vi "Debug Settings FG.vi"(8 "error in (no error)":errorcluster, 10 "Debug Settings In":T2, 11 "Operation":T1) -> (0 "error out":errorcluster, 2 "Debug Settings Out":T2)   [LabVIEW 2013]
uses:
  Debug Settings Cluster.ctl
  Debug Settings FG Enum.ctl
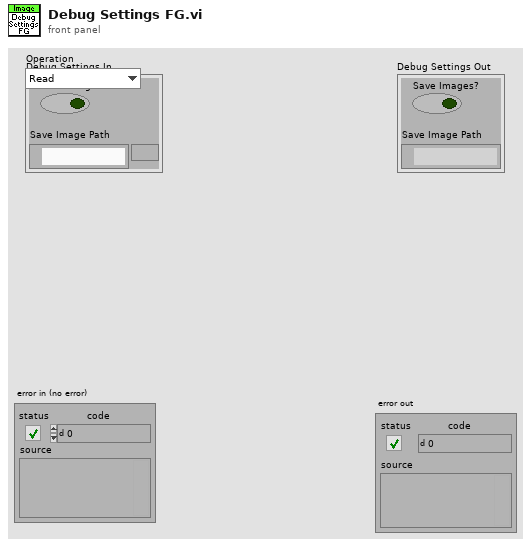
[diagram p1: front panel]
types:
  T1 = typedef "Debug Settings FG Enum.ctl" = enum16{"Read", "Write"}
  T2 = typedef "Debug Settings Cluster.ctl" = cluster{"Save Images?":bool, "Save Image Path":path}
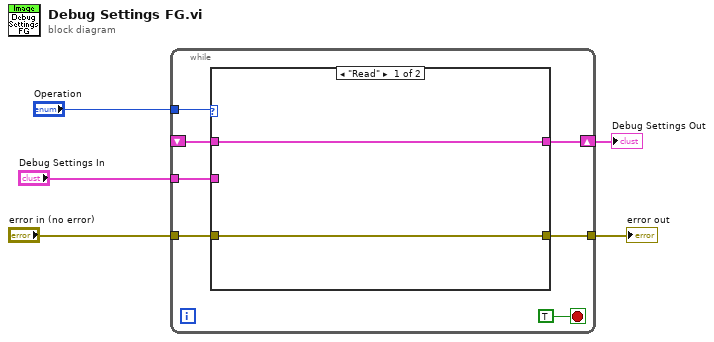
[diagram p0: block diagram]
diagram:
  n1 = while {
    tunnel: "Operation" -> [w11]
    tunnel: "Debug Settings In" -> [w10]
    shift-right: [w9] -> w3
    shift-left: _ -> [w8]
    tunnel: [w7] -> w2
    tunnel: "error in (no error)" -> [w6]
    stop <- TRUE stop-if-true
    n2 = case shown="\"Read\"" w11 {
      tunnel: w10 -> [_ w16]
      tunnel: [w14 w16] -> w9
      tunnel: w8 -> [w14 _]
      tunnel: [w13 w15] -> w7
      tunnel: w6 -> [w13 w15]
      frame "Read" {
      }
      frame "Write" {
      }
    }
  }
  "Debug Settings Out" <- w3
  "error out" <- w2
